vi "CTRE_PigeonIMU_ConfigSlot.vi"(6 "timeoutMs":i32=50, 8 "error in":errorcluster, 10 "Pigeon Config Parameters":T1, 11 "PigeonIMUDevRef":T3={"DeviceStatus"={"status"=FALSE, "code"=0, "source"=""}, "Device Number"=0, "Type"=352321536, "Device ID"=0, "Handle"=0, "UsageFrame"=0, "Library Path"=path ""} {"Type" items=["CAN"=352321536, "TalonSRX"=33554432]}) -> (0 "error out":errorcluster, 3 "PigeonIMUDevRef":T3={"DeviceStatus"={"status"=FALSE, "code"=0, "source"=""}, "Device Number"=0, "Type"=352321536, "Device ID"=0, "Handle"=0, "UsageFrame"=0, "Library Path"=path ""} {"Type" items=["CAN"=352321536, "TalonSRX"=33554432]})   [LabVIEW 2020]
doc: "Configures all persistant settings\n\n<b> Pigeon Config Parameters </b> Cluster of all the persistant settings"
uses:
  <vilib>/Rock Robotics/WPI/ThirdParty/Phoenix-LabVIEW/Pigeon IMU/CTRE_PigeonIMU_DeviceRef.ctl
  <vilib>/Rock Robotics/WPI/ThirdParty/Phoenix-LabVIEW/Pigeon IMU/CTRE_PigeonIMU_ConnectionType.ctl
  <vilib>/Rock Robotics/WPI/ThirdParty/Phoenix-LabVIEW/Pigeon IMU/CTRE_PigeonIMU_Configurables.ctl
  <vilib>/Rock Robotics/WPI/ThirdParty/Phoenix-LabVIEW/Controls/CTRE_Phoenix_CustomParamConfiguration.ctl
panel:
  in  "Force Write":bool
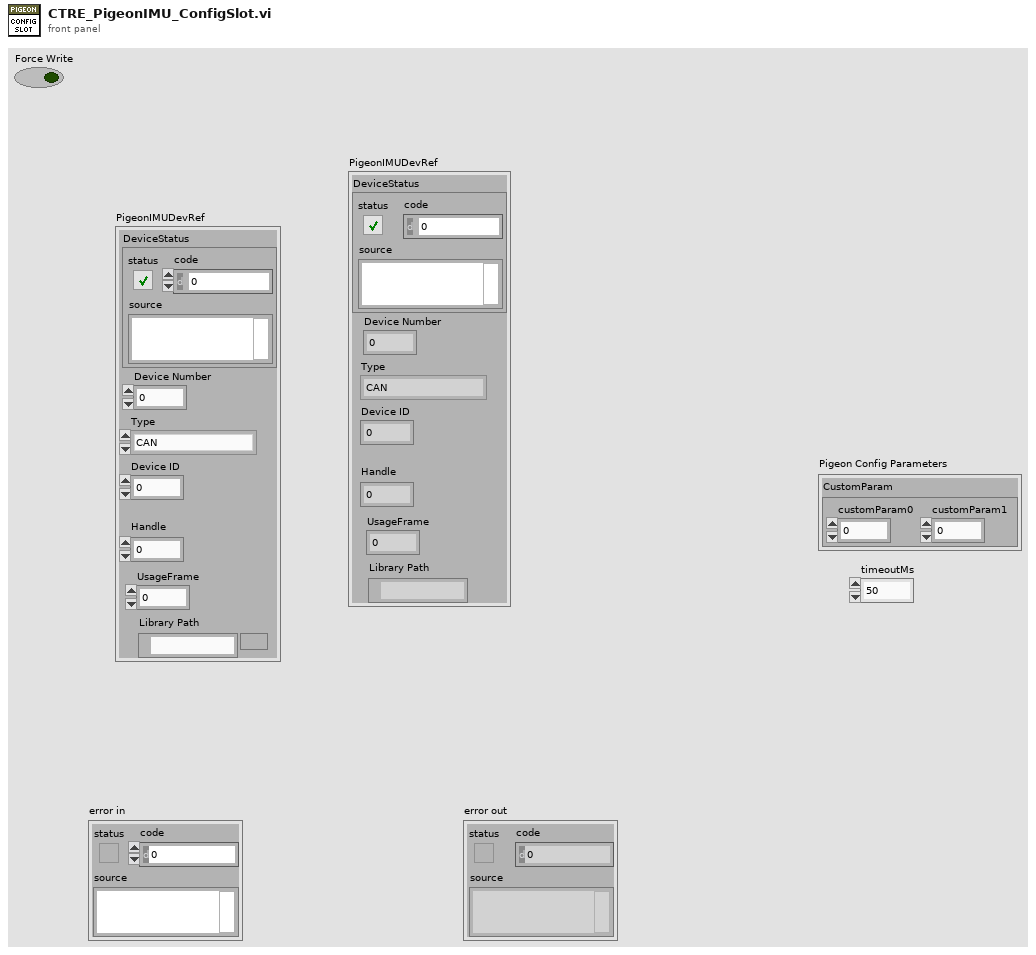
[diagram p1: front panel]
types:
  T1 = typedef "CTRE_PigeonIMU_Configurables.ctl" = cluster{"CustomParam":T2}
  T2 = typedef "CTRE_Phoenix_CustomParamConfiguration.ctl" = cluster{"customParam0":i32, "customParam1":i32}
  T3 = typedef "CTRE_PigeonIMU_DeviceRef.ctl" = cluster{"DeviceStatus":errorcluster, "Device Number":u8, "Type":T4, "Device ID":u32, "Handle":u64, "UsageFrame":u32, "Library Path":path}
  T4 = typedef "CTRE_PigeonIMU_ConnectionType.ctl" = u32
  T5 = cluster{"CustomParam":cluster{"customParam0":bool, "customParam1":bool}}
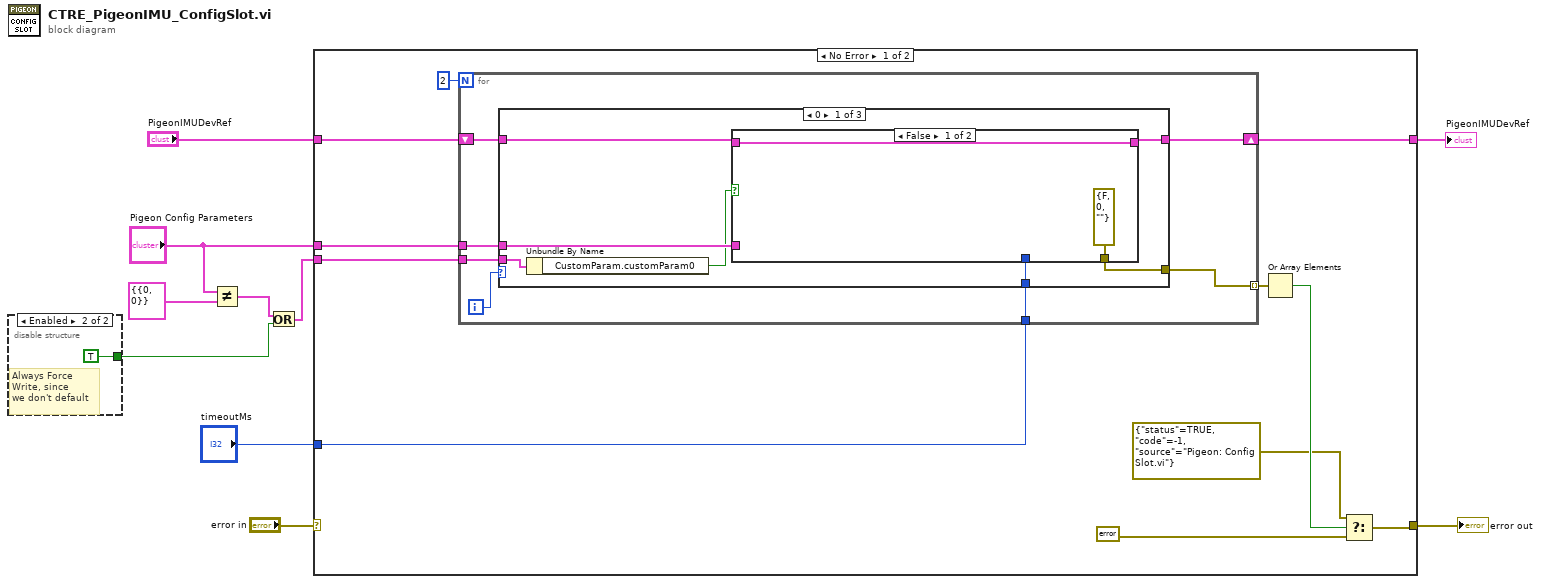
[diagram p0: block diagram]
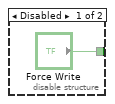
[diagram p2: hidden frame]
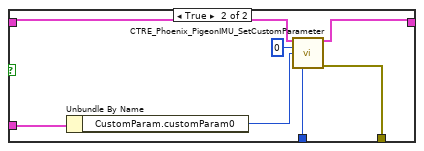
[diagram p3: hidden frame]
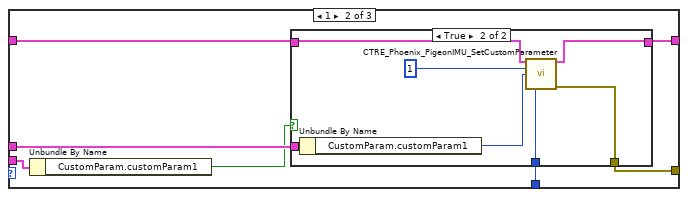
[diagram p4: hidden frame]
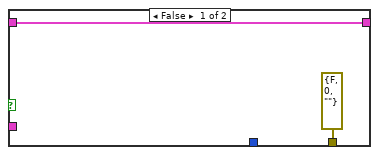
[diagram p5: hidden frame]
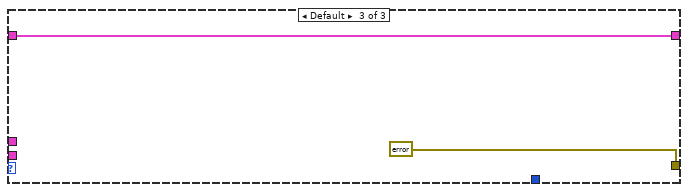
[diagram p6: hidden frame]
diagram:
  n1 = disable-structure shown="Enabled" {
    disable-tunnel: ["Force Write" TRUE ("Force Write")] -> w2
    frame Disabled {
    }
    frame Enabled {
      # "Always Force\nWrite, since\nwe don't default"
    }
  }
  n2 = Not Equal?(x="Pigeon Config Parameters", y=T1 {"CustomParam"={"customParam0"=0, "customParam1"=0}}) -> (x != y?=w3:T5)
  n3 = Or(x=w3, y=w2) -> (x .or. y?=w1:T5)
  n4 = case shown="No Error" "error in" {
    selector: "error in" -> [_ w66]
    tunnel: [w18 w66] -> w9
    tunnel: "PigeonIMUDevRef" -> [w23 w65]
    tunnel: "timeoutMs" -> [w20 _]
    tunnel: [w22 w65] -> w6
    tunnel: "Pigeon Config Parameters" -> [w21 _]
    tunnel: w1 -> [w13 _]
    frame No Error {
      n5 = for {
        N: 2 -> [_]
        shift-right: [w28] -> w22
        shift-left: w23 -> [w29]
        tunnel: w21 -> [w27]
        tunnel: [w26] -> w19 mode=indexing
        tunnel: w20 -> [w25]
        tunnel: w13 -> [w24]
        i -> [w30]
        n6 = case shown="0" w30 {
          tunnel: w29 -> [w37 w53 w64]
          tunnel: [w36 w52 w64] -> w28
          tunnel: w27 -> [w35 w51 _]
          tunnel: [w34 w50 errorcluster {"status"=FALSE, "code"=0, "source"=""} ("error out")] -> w26
          tunnel: w25 -> [w33 w49 _]
          tunnel: w24 -> [w32 w48 _]
          frame 0 {
            n7 = Unbundle By Name(w32) -> ("CustomParam.customParam0"=w31:bool)
            n8 = case shown="False" w31 {
              tunnel: w37 -> [w39 w46]
              tunnel: [w39 w45] -> w36
              tunnel: w35 -> [_ w43]
              tunnel: [errorcluster {"status"=FALSE, "code"=0, "source"=""} ("error out") w41] -> w34
              tunnel: w33 -> [_ w40]
              frame False {
              }
              frame True {
                n9 = Unbundle By Name(w43) -> ("CustomParam.customParam0"=w42:i32)
                n10 = call <vilib>:"CTRE_Phoenix_PigeonIMU_SetCustomParameter.vi"("PigeonIMUDevRef"=w46, "paramIdx"=u32 0, "value"=w42, "timeoutMs"=w40) -> ("PigeonIMUDevRef"=w45:T3, "error out"=w41:errorcluster)  [unwired: 10 in]
              }
            }
          }
          frame 1 {
            n11 = Unbundle By Name(w48) -> ("CustomParam.customParam1"=w47:bool)
            n12 = case shown="True" w47 {
              tunnel: w53 -> [w55 w62]
              tunnel: [w55 w61] -> w52
              tunnel: w51 -> [_ w59]
              tunnel: [errorcluster {"status"=FALSE, "code"=0, "source"=""} ("error out") w57] -> w50
              tunnel: w49 -> [_ w56]
              frame False {
              }
              frame True {
                n13 = Unbundle By Name(w59) -> ("CustomParam.customParam1"=w58:i32)
                n14 = call <vilib>:"CTRE_Phoenix_PigeonIMU_SetCustomParameter.vi"("PigeonIMUDevRef"=w62, "paramIdx"=u32 1, "value"=w58, "timeoutMs"=w56) -> ("PigeonIMUDevRef"=w61:T3, "error out"=w57:errorcluster)  [unwired: 10 in]
              }
            }
          }
          frame Default {
          }
        }
      }
      n15 = Or Array Elements(Boolean array=w19) -> (logical OR=w16:bool)
      n16 = Select(t=errorcluster {"status"=TRUE, "code"=-1, "source"="Pigeon: Config Slot.vi"} ("error out"), s=w16, f=errorcluster {"status"=FALSE, "code"=0, "source"=""} ("error out")) -> (s? t:f=w18:errorcluster)
    }
    frame Error {
    }
  }
  "error out" <- w9
  "PigeonIMUDevRef" <- w6
